vi "总氮总磷质控流程.vi"(0 "队列输入TP":refnum<queue>, 5 "总氮量程切换":enum32{"H", "L", "AUTO"}(ring)=enum."AUTO", 7 "总磷量程切换":enum32{"H", "L", "AUTO"}(ring)=enum."AUTO", 9 "总磷":bool, 11 "总氮":bool) -> (4 "布尔":bool, 6 "总磷中断报警":bool, 8 "总氮中断报警":bool)   [LabVIEW 2016, in "质控单元.lvlib"]
panel:
  out "总磷":bool
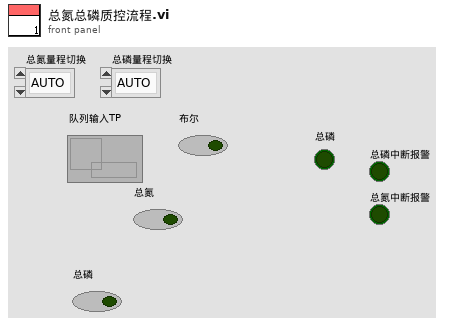
[diagram p1: front panel]
types:
  T1 = enum16{"待机", "启动氨氮水样", "氨氮测量中", "启动氨氮加标", "启动氨氮加标回收", "氨氮加标回收测量中", "启动总氮水样", "总氮测量中", "启动总氮加标", "启动总氮加标回收", "总氮加标回收测量中", "启动总磷水样", "总磷水样测量中", "启动总磷加标", "启动总磷加标回收", "总磷加标回收测量中", "结束"}
  T2 = cluster{"时间标识":timestamp, "设备":string, "日志信息":string}
  T3 = cluster{"站号":u16, "量程切换":enum32{"H", "L", "AUTO"}, "控制命令":enum16{"启动测量", "标样核查", "零点核查", "跨度核查", "空白测试", "平行样测试", "加标回收", "空白校准", "标样校准", "初始化（清洗）", "停止测试", "仪器重启", "校时", "模式设置", "测量间隔设置"}, "模式设置":enum16{"待机", "连续模式", "周期模式", "定点模式", "受控模式", "手动模式"}, "测量间隔":u16}
  T4 = cluster{"系统时间":timestamp, "工作状态":enum16{"空闲", "水样测试", "标样核查", "零点核查", "跨度核查", "空白测试", "平行样测试", "加标回收", "空白校准", "标样校准", "初始化（清洗）"}, "测量模式":enum16{"待机", "连续模式", "周期模式", "定点模式", "受控模式", "手动模式"}, "告警代码":enum16{"无告警", "缺试剂告警", "缺水样告警", "缺蒸馏水告警", "缺标液告警", "仪表漏液告警", "标定异常告警", "超量程告警", "加热异常", "低试剂预警", "超上限告警", "超下限告警", "仪表内部其他异常", "滴定异常告警", "电极异常告警", "量程切换告警", "参数设置告警", "PH电极电位异常", "电导率电极异常", "浊度光度异常", "溶解氧电极异常", "溶解氧光强异常", "温度异常告警", "PH异常告警", "溶解氧异常告警", "电导率异常告警", "浊度异常告警", "叶绿素异常告警", "藻密度异常告警", "蓝绿藻异常告警", "ORP异常告警", "氨氮异常告警", "清洁刷异常告警", "SD卡异常告警", "蓝牙异常告警", "Wifi异常告警", "流程异常告警"}, "故障代码":enum16{"无故障", "电机故障", "温度故障", "通讯故障", "滴定故障"}, "日志代码":u16, "软件版本":u16, "F0":sgl, "F1":sgl, "F2":sgl, "F3":sgl, "T":sgl, "H":sgl, "id":u16, "flowid":u16, "量程":u16}
  T5 = enum16{"空闲", "水样测试", "标样核查", "零点核查", "跨度核查", "空白测试", "平行样测试", "加标回收", "空白校准", "标样校准", "初始化（清洗）"}
  T6 = cluster{"因子编码":u32, "单位":u16, "标样参考值":sgl, "水样数据时间":timestamp, "水样实测值":sgl, "水样数据标识":string, "标样数据时间":timestamp, "标样实测值":sgl, "标样数据标识":string, "空白数据时间":timestamp, "空白实测值":sgl, "空白数据标识":string, "零点核查数据时间":timestamp, "零点核查实测值":sgl, "零点核查数据标识":string, "跨度核查数据时间":timestamp, "跨度核查实测值":sgl, "跨度核查数据标识":string, "加标回收数据时间":timestamp, "加标回收实测值":sgl, "加标回收数据标识":string, "平行样数据时间":timestamp, "平行样实测值":sgl, "平行样数据标识":string}
  T7 = cluster{"量程":dbl, "检出限":dbl, "加标前水样浓度":dbl, "加标后水样浓度":dbl, "加标水杯定容体积":dbl, "加标母液浓度":dbl, "加标体积":dbl, "加标回收率":dbl}
  T8 = cluster{"因子编码":u32, "单位":u16, "标样参考值":sgl, "水样数据时间":timestamp, "水样实测值":sgl, "水样数据标识":string, "标样数据时间":timestamp, "标样实测值":sgl, "标样数据标识":string, "空白数据时间":timestamp, "空白实测值":sgl, "空白数据标识":string, "零点核查数据时间":timestamp, "零点核查实测值":sgl, "零点核查数据标识":string, "跨度核查数据时间":timestamp, "跨度核查实测值":sgl, "跨度核查数据标识":string, "加标回收数据时间":timestamp, "加标回收实测值":sgl, "加标回收数据标识":string, "平行样数据时间":timestamp, "平行样实测值":sgl, "平行样数据标识":string, "F0":sgl, "F1":sgl, "F2":sgl, "F3":sgl, "F4":sgl, "F5":sgl, "F6":sgl, "F7":sgl, "温度":sgl, "湿度":sgl, "X值":sgl}
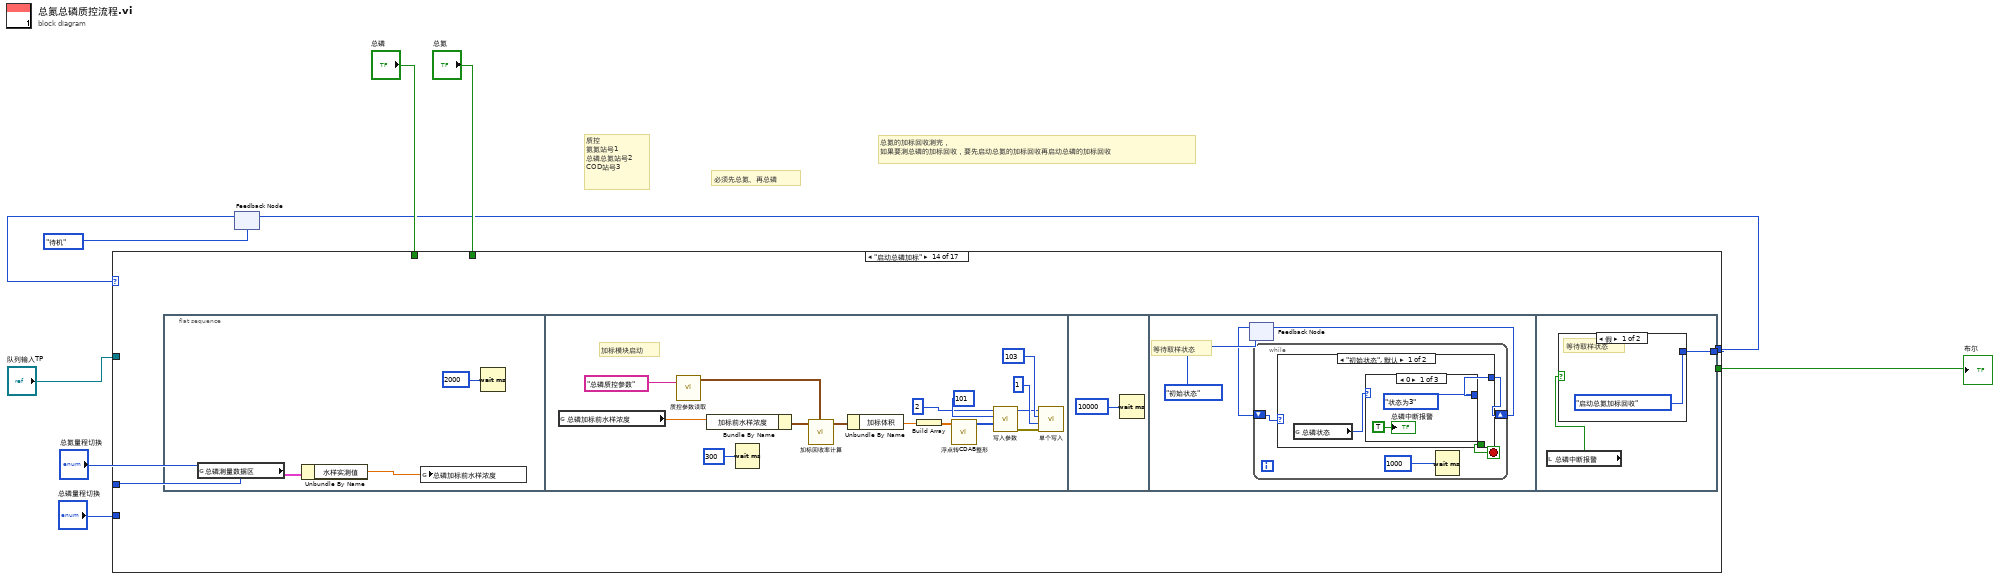
[diagram p0: block diagram]
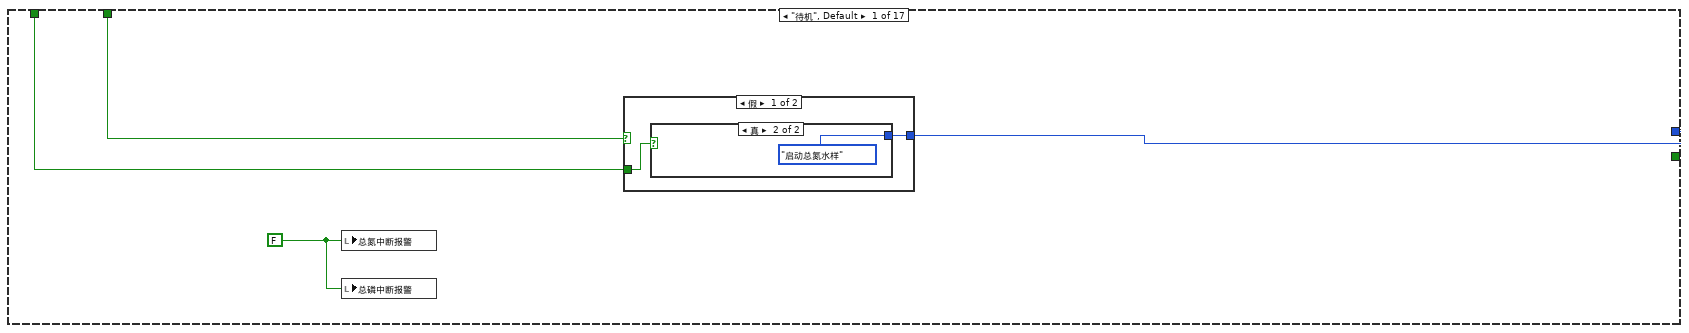
[diagram p2: hidden frame]
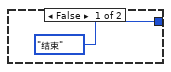
[diagram p3: hidden frame]
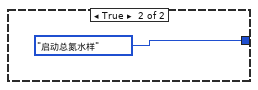
[diagram p4: hidden frame]
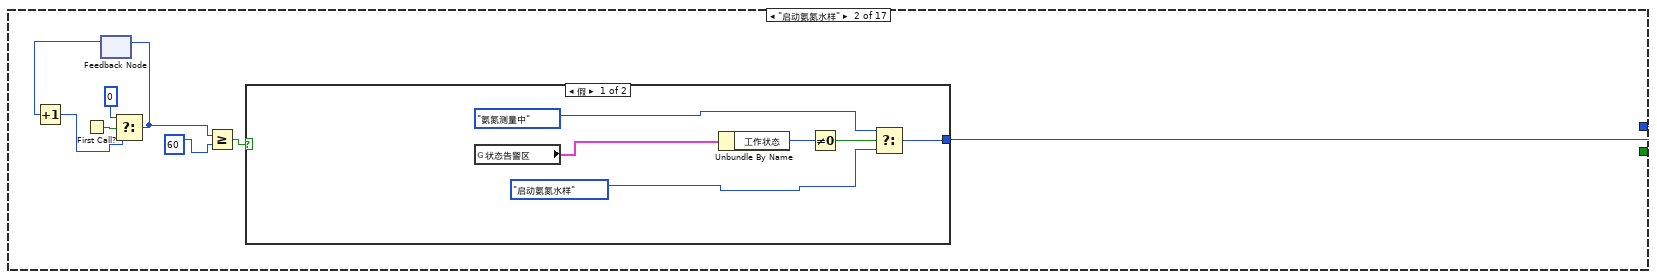
[diagram p5: hidden frame]
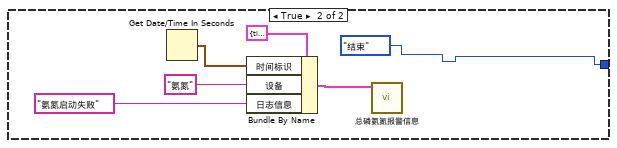
[diagram p6: hidden frame]
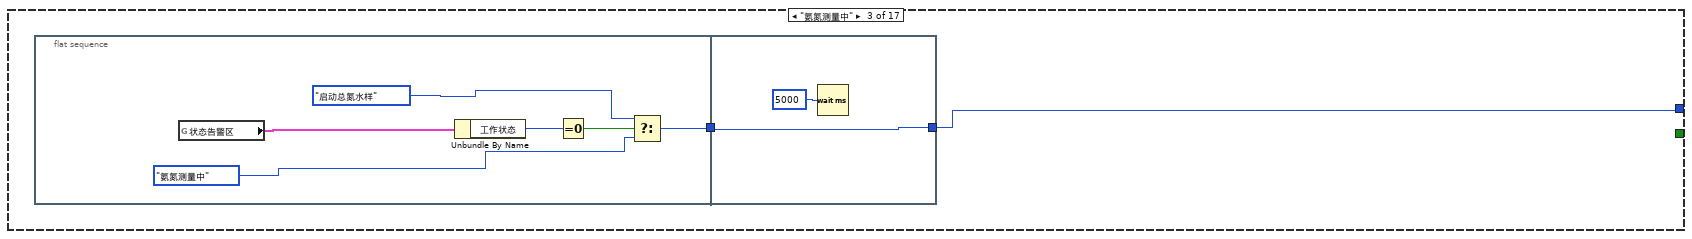
[diagram p7: hidden frame]
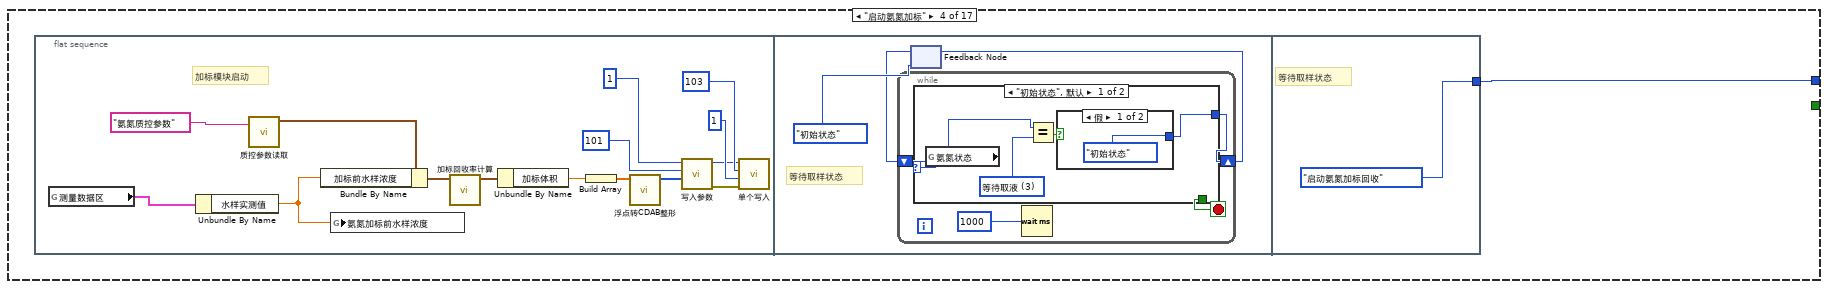
[diagram p8: hidden frame]
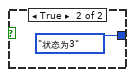
[diagram p9: hidden frame]
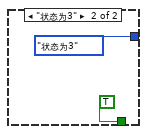
[diagram p10: hidden frame]
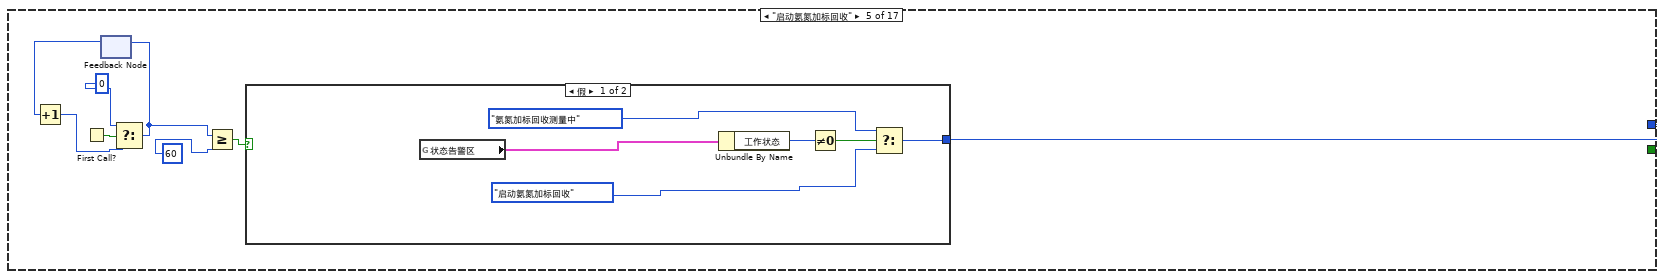
[diagram p11: hidden frame]
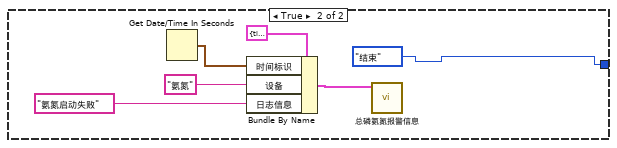
[diagram p12: hidden frame]
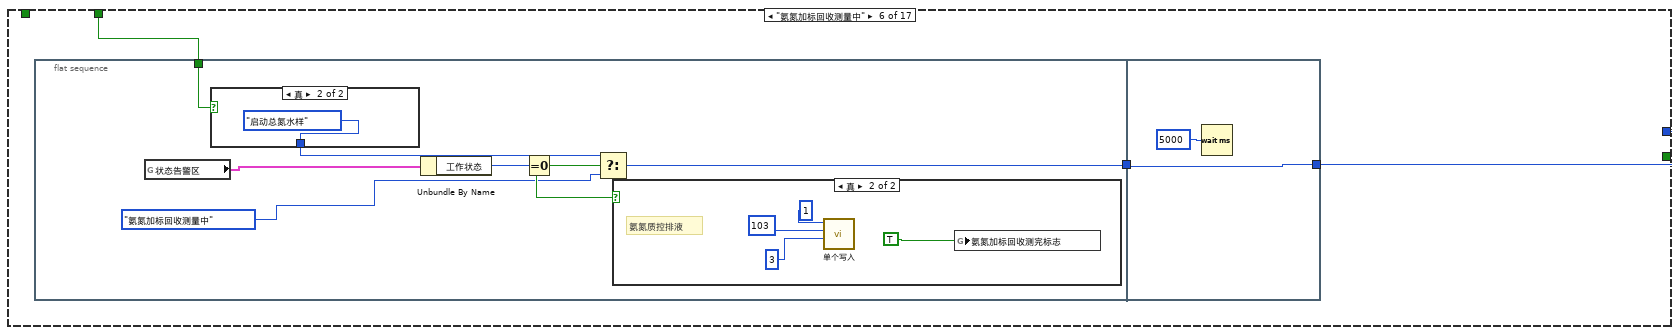
[diagram p13: hidden frame]
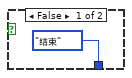
[diagram p14: hidden frame]
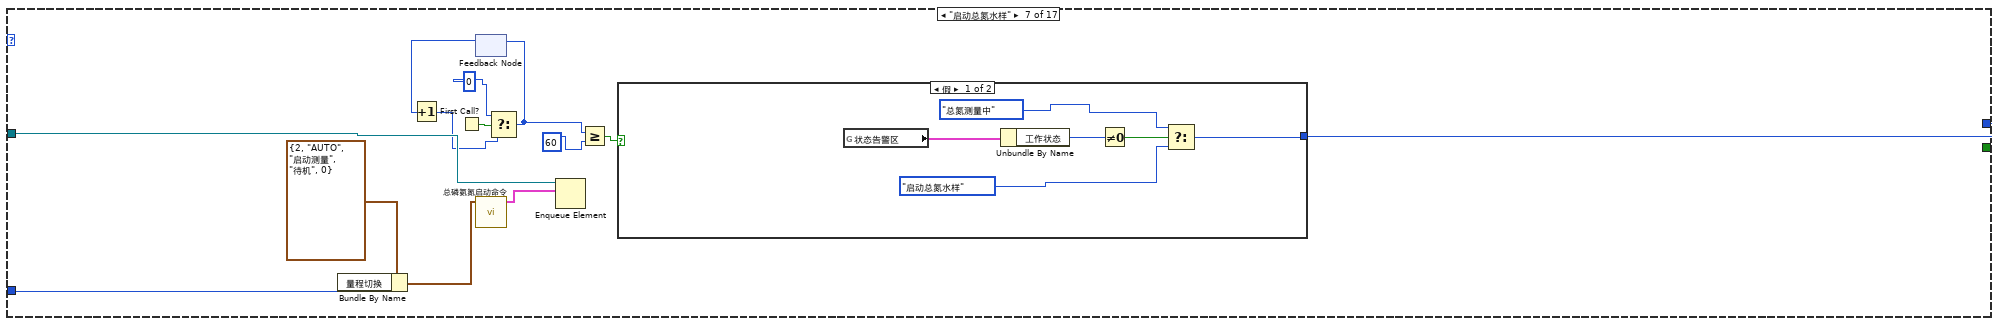
[diagram p16: hidden frame]
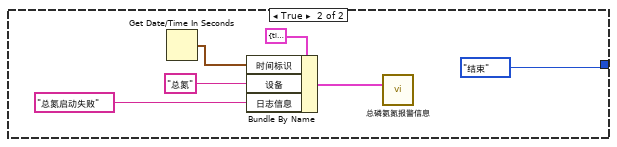
[diagram p17: hidden frame]
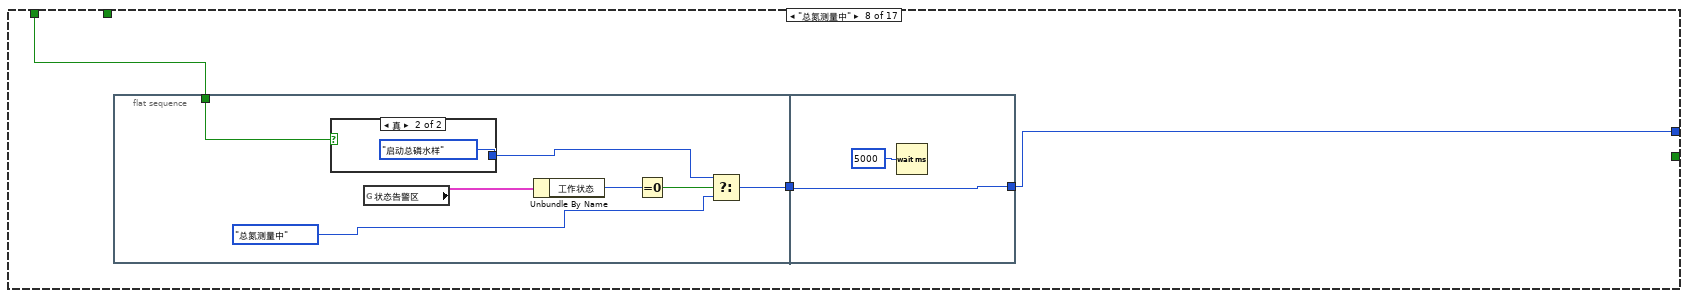
[diagram p18: hidden frame]
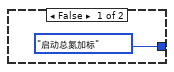
[diagram p19: hidden frame]
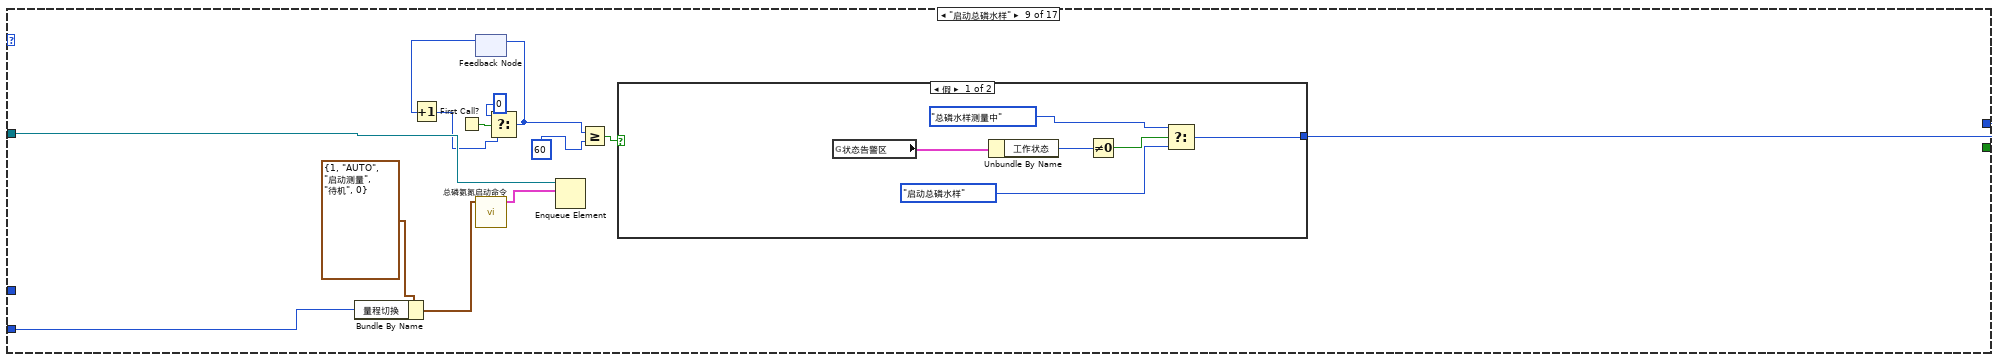
[diagram p20: hidden frame]
diagram:
  # "总氮的加标回收测完，\n如果要测总磷的加标回收，要先启动总氮的加标回收再启动总磷的加标回收"
  # "质控\n氨氮站号1   \n总磷总氮站号2\nCOD站号3"
  # "必须先总氮、再总磷"
  n1 = feedback #1(T1."待机") -> (w5:T1)
  n2 = case shown="\"启动总磷加标\"" w5 {
    tunnel: [w13 w26 w40 w49 w80 w100 w129 w144 w168 w184 w196 w238 w261 w290 w334 w356 T1."结束"] -> w3
    tunnel: "队列输入TP" -> [_ _ _ _ _ _ w130 _ w169 _ _ w240 _ _ w335 _ _]
    tunnel: [_ _ _ _ _ _ _ _ _ _ _ _ _ _ _ _ TRUE] -> w8
    tunnel: "总磷" -> [w12 _ _ _ _ _ _ w143 _ _ _ _ w262 _ _ _ _]
    tunnel: "总氮" -> [w11 _ _ _ _ w101 _ _ _ w182 _ _ w260 _ _ _ _]
    tunnel: "总氮量程切换" -> [_ _ _ _ _ _ w118 _ _ _ _ w235 _ _ _ _ _]
    tunnel: "总磷量程切换" -> [_ _ _ _ _ _ _ _ w157 _ _ _ _ _ w330 _ _]
    frame "待机", Default {
      w10 = FALSE ("总氮中断报警")
      n3 = local write "总氮中断报警"(w10) -> ()
      n4 = local write "总磷中断报警"(w10) -> ()
      n5 = case shown="假" w11 {
        tunnel: w12 -> [w14 _]
        tunnel: [w15 T1."启动总氮水样"] -> w13
        frame False {
          n6 = case shown="真" w14 {
            tunnel: [T1."结束" T1."启动总氮水样"] -> w15
            frame False {
            }
            frame True {
            }
          }
        }
        frame True {
        }
      }
    }
    frame "启动氨氮水样" {
      n7 = First Call?() -> (First Call?: T/F=w24:bool)
      n8 = feedback #2() -> (w23:i32)  [unwired: 1 in]
      n9 = Increment(x=w23) -> (x+1=w22:i32)
      n10 = Select(t=0, s=w24, f=w22) -> (s? t:f=w21:i32)
      n11 = feedback-in #2(w21) -> ()
      n12 = Greater Or Equal?(x=w21, y=60) -> (x >= y?=w19:bool)
      n13 = case shown="假" w19 {
        tunnel: [w30 T1."结束"] -> w26
        frame False {
          n14 = global read "VAR总磷氨氮全局变量.vi" "状态告警区"() -> (w27:T4)
          n15 = Unbundle By Name(w27) -> ("工作状态"=w32:T5)
          n16 = Not Equal To 0?(x=w32) -> (x != 0?=w31:bool)
          n17 = Select(t=T1."氨氮测量中", s=w31, f=T1."启动氨氮水样") -> (s? t:f=w30:T1)
        }
        frame True {
          n18 = Get Date/Time In Seconds() -> (seconds since 1Jan1904=w38:timestamp)
          n19 = Bundle By Name(cluster=T2 {"时间标识"=timestamp(0 s since 1904-01-01), "设备"="", "日志信息"=""} ("data in"), "时间标识"=w38, "设备"="氨氮", "日志信息"="氨氮启动失败") -> (w34:T2)
          n20 = call "总磷氨氮报警信息.vi"("data in"=w34) -> ()  [unwired: 11 in]
        }
      }
    }
    frame "氨氮测量中" {
      n21 = flat-sequence {
        tunnel: [w45] -> w39
        tunnel: [w48] -> w40
        tunnel: w39 -> [w48]
        frame #0 {
          n22 = global read "VAR总磷氨氮全局变量.vi" "状态告警区"() -> (w41:T4)
          n23 = Unbundle By Name(w41) -> ("工作状态"=w46:T5)
          n24 = Equal To 0?(x=w46) -> (x = 0?=w44:bool)
          n25 = Select(t=T1."启动总氮水样", s=w44, f=T1."氨氮测量中") -> (s? t:f=w45:T1)
        }
        frame #1 {
          n26 = Wait (ms)(milliseconds to wait=u32 5000 ("等待时间（毫秒）")) -> ()  [unwired: 1 out]
        }
      }
    }
    frame "启动氨氮加标" {
      n27 = flat-sequence {
        tunnel: [T1."启动氨氮加标回收"] -> w49
        frame #0 {
          w53 = u16 1 ("value")
          # "加标模块启动"
          n28 = global read "VAR总磷氨氮全局变量.vi" "测量数据区"() -> (w50:T6)
          n29 = Unbundle By Name(w50) -> ("水样实测值"=w51:sgl)
          n30 = call "质控参数读取.vi"("section"="氨氮质控参数") -> ("参数"=w61:T7)  [unwired: 9 in, 1 out]
          n31 = Bundle By Name(cluster=w61, "加标前水样浓度"=w51) -> (w62:T7)
          n32 = global write "水样浓度全局.vi" "氨氮加标前水样浓度"(w51) -> ()
          n33 = call "加标回收率计算.vi"("参数"=w62) -> ("参数 out"=w60:T7)  [unwired: 10 in]
          n34 = Unbundle By Name(w60) -> ("加标体积"=w52:dbl)
          n35 = Build Array(w52) -> (w59:dbl[])
          n36 = call "浮点转CDAB整形.vi"("浮点数"=w59) -> ("CDAB整形输出"=w54:u16[])  [unwired: 10 in]
          n37 = call "写入参数.vi"("values"=w54, "starting address"=u16 101, "Slave ID"=w53) -> ("error out"=w58:errorcluster)  [unwired: 8 in]
          n38 = call "单个写入.vi"("Error in"=w58, "value"=u16 1, "address"=u16 103, "Slave ID"=w53) -> ()  [unwired: 7 in, 1 out]
        }
        frame #1 {
          # "等待取样状态"
          n39 = feedback #3(enum16{"初始状态", "状态为3"}."初始状态") -> (w65:enum16{"初始状态", "状态为3"})
          n40 = while {
            shift-right: [w69] -> w64
            shift-left: w65 -> [w70]
            stop <- w68 stop-if-true
            n41 = case shown="\"初始状态\", 默认" w70 {
              tunnel: [w72 enum16{"初始状态", "状态为3"}."状态为3"] -> w69
              tunnel: [_ TRUE] -> w68
              frame "初始状态", Default {
                w71 = u16 3 items=["待机", "润洗", "进样", "等待取液", "排液"] ("氨氮状态")
                n42 = global read "氨氮加标回收状态全局变量.vi" "氨氮状态"() -> (w74:u16)
                n43 = Equal?(x=w74, y=w71) -> (x = y?=w73:bool)
                n44 = case shown="假" w73 {
                  tunnel: [enum16{"初始状态", "状态为3"}."初始状态" enum16{"初始状态", "状态为3"}."状态为3"] -> w72
                  frame False {
                  }
                  frame True {
                  }
                }
              }
              frame "状态为3" {
              }
            }
            n45 = Wait (ms)(milliseconds to wait=u32 1000 ("等待时间（毫秒）")) -> ()  [unwired: 1 out]
          }
          n46 = feedback-in #3(w64) -> ()
        }
        frame #2 {
          # "等待取样状态"
        }
      }
    }
    frame "启动氨氮加标回收" {
      n47 = First Call?() -> (First Call?: T/F=w86:bool)
      n48 = feedback #4() -> (w85:i32)  [unwired: 1 in]
      n49 = Increment(x=w85) -> (x+1=w84:i32)
      n50 = Select(t=0, s=w86, f=w84) -> (s? t:f=w83:i32)
      n51 = feedback-in #4(w83) -> ()
      n52 = Greater Or Equal?(x=w83, y=60) -> (x >= y?=w81:bool)
      n53 = case shown="假" w81 {
        tunnel: [w91 T1."结束"] -> w80
        frame False {
          n54 = global read "VAR总磷氨氮全局变量.vi" "状态告警区"() -> (w88:T4)
          n55 = Unbundle By Name(w88) -> ("工作状态"=w93:T5)
          n56 = Not Equal To 0?(x=w93) -> (x != 0?=w92:bool)
          n57 = Select(t=T1."氨氮加标回收测量中", s=w92, f=T1."启动氨氮加标回收") -> (s? t:f=w91:T1)
        }
        frame True {
          n58 = Get Date/Time In Seconds() -> (seconds since 1Jan1904=w99:timestamp)
          n59 = Bundle By Name(cluster=T2 {"时间标识"=timestamp(0 s since 1904-01-01), "设备"="", "日志信息"=""} ("data in"), "时间标识"=w99, "设备"="氨氮", "日志信息"="氨氮启动失败") -> (w95:T2)
          n60 = call "总磷氨氮报警信息.vi"("data in"=w95) -> ()  [unwired: 11 in]
        }
      }
    }
    frame "氨氮加标回收测量中" {
      n61 = flat-sequence {
        tunnel: [w108] -> w102
        tunnel: w101 -> [w105]
        tunnel: [w117] -> w100
        tunnel: w102 -> [w117]
        frame #0 {
          n62 = global read "VAR总磷氨氮全局变量.vi" "状态告警区"() -> (w103:T4)
          n63 = case shown="真" w105 {
            tunnel: [T1."结束" T1."启动总氮水样"] -> w107
            frame False {
            }
            frame True {
            }
          }
          n64 = Unbundle By Name(w103) -> ("工作状态"=w109:T5)
          n65 = Equal To 0?(x=w109) -> (x = 0?=w106:bool)
          n66 = Select(t=w107, s=w106, f=T1."氨氮加标回收测量中") -> (s? t:f=w108:T1)
          n67 = case shown="真" w106 {
            frame False {
            }
            frame True {
              # "氨氮质控排液"
              n68 = call "单个写入.vi"("value"=u16 3, "address"=u16 103, "Slave ID"=u8 1) -> ()  [unwired: 8 in, 1 out]
              n69 = global write "质控测完标志全局 1.vi" "氨氮加标回收测完标志"(TRUE) -> ()
            }
          }
        }
        frame #1 {
          n70 = Wait (ms)(milliseconds to wait=u32 5000 ("等待时间（毫秒）")) -> ()  [unwired: 1 out]
        }
      }
    }
    frame "启动总氮水样" {
      n71 = Bundle By Name(cluster=T3 {"站号"=2, "量程切换"=enum."AUTO", "控制命令"=enum."启动测量", "模式设置"=enum."待机", "测量间隔"=0} ("参数"), "量程切换"=w118) -> (w119:T3)
      n72 = First Call?() -> (First Call?: T/F=w127:bool)
      n73 = feedback #5() -> (w126:i32)  [unwired: 1 in]
      n74 = Increment(x=w126) -> (x+1=w125:i32)
      n75 = call "总磷氨氮启动命令.vi"("参数"=w119) -> ("启动命令"=w121:cluster{"命令":string, "data":variant})  [unwired: 10 in]
      n76 = Select(t=0, s=w127, f=w125) -> (s? t:f=w124:i32)
      n77 = feedback-in #5(w124) -> ()
      n78 = Enqueue Element(queue=w130, element=w121) -> ()  [unwired: 2 in, 3 out]
      n79 = Greater Or Equal?(x=w124, y=60) -> (x >= y?=w122:bool)
      n80 = case shown="假" w122 {
        tunnel: [w133 T1."结束"] -> w129
        frame False {
          n81 = global read "VAR总磷氨氮全局变量.vi" "状态告警区"() -> (w134:T4)
          n82 = Unbundle By Name(w134) -> ("工作状态"=w135:T5)
          n83 = Not Equal To 0?(x=w135) -> (x != 0?=w136:bool)
          n84 = Select(t=T1."总氮测量中", s=w136, f=T1."启动总氮水样") -> (s? t:f=w133:T1)
        }
        frame True {
          n85 = Get Date/Time In Seconds() -> (seconds since 1Jan1904=w142:timestamp)
          n86 = Bundle By Name(cluster=T2 {"时间标识"=timestamp(0 s since 1904-01-01), "设备"="", "日志信息"=""} ("data in"), "时间标识"=w142, "设备"="总氮", "日志信息"="总氮启动失败") -> (w138:T2)
          n87 = call "总磷氨氮报警信息.vi"("data in"=w138) -> ()  [unwired: 11 in]
        }
      }
    }
    frame "总氮测量中" {
      n88 = flat-sequence {
        tunnel: [w150] -> w145
        tunnel: w143 -> [w146]
        tunnel: [w156] -> w144
        tunnel: w145 -> [w156]
        frame #0 {
          n89 = case shown="真" w146 {
            tunnel: [T1."启动总氮加标" T1."启动总磷水样"] -> w148
            frame False {
            }
            frame True {
            }
          }
          n90 = global read "VAR总磷氨氮全局变量.vi" "状态告警区"() -> (w151:T4)
          n91 = Unbundle By Name(w151) -> ("工作状态"=w152:T5)
          n92 = Equal To 0?(x=w152) -> (x = 0?=w149:bool)
          n93 = Select(t=w148, s=w149, f=T1."总氮测量中") -> (s? t:f=w150:T1)
        }
        frame #1 {
          n94 = Wait (ms)(milliseconds to wait=u32 5000 ("等待时间（毫秒）")) -> ()  [unwired: 1 out]
        }
      }
    }
    frame "启动总磷水样" {
      n95 = Bundle By Name(cluster=T3 {"站号"=1, "量程切换"=enum."AUTO", "控制命令"=enum."启动测量", "模式设置"=enum."待机", "测量间隔"=0} ("参数"), "量程切换"=w157) -> (w158:T3)
      n96 = First Call?() -> (First Call?: T/F=w166:bool)
      n97 = feedback #6() -> (w165:i32)  [unwired: 1 in]
      n98 = Increment(x=w165) -> (x+1=w164:i32)
      n99 = call "总磷氨氮启动命令.vi"("参数"=w158) -> ("启动命令"=w160:cluster{"命令":string, "data":variant})  [unwired: 10 in]
      n100 = Select(t=0, s=w166, f=w164) -> (s? t:f=w163:i32)
      n101 = feedback-in #6(w163) -> ()
      n102 = Enqueue Element(queue=w169, element=w160) -> ()  [unwired: 2 in, 3 out]
      n103 = Greater Or Equal?(x=w163, y=60) -> (x >= y?=w161:bool)
      n104 = case shown="假" w161 {
        tunnel: [w172 T1."结束"] -> w168
        frame False {
          n105 = global read "VAR总磷氨氮全局变量.vi" "状态告警区"() -> (w173:T4)
          n106 = Unbundle By Name(w173) -> ("工作状态"=w174:T5)
          n107 = Not Equal To 0?(x=w174) -> (x != 0?=w175:bool)
          n108 = Select(t=T1."总磷水样测量中", s=w175, f=T1."启动总磷水样") -> (s? t:f=w172:T1)
        }
        frame True {
          n109 = Get Date/Time In Seconds() -> (seconds since 1Jan1904=w181:timestamp)
          n110 = Bundle By Name(cluster=T2 {"时间标识"=timestamp(0 s since 1904-01-01), "设备"="", "日志信息"=""} ("data in"), "时间标识"=w181, "设备"="总磷", "日志信息"="总磷启动失败") -> (w177:T2)
          n111 = call "总磷氨氮报警信息.vi"("data in"=w177) -> ()  [unwired: 11 in]
        }
      }
    }
    frame "总磷水样测量中" {
      n112 = flat-sequence {
        tunnel: [w189] -> w183
        tunnel: w182 -> [w186]
        tunnel: [w195] -> w184
        tunnel: w183 -> [w195]
        frame #0 {
          n113 = case shown="真" w186 {
            tunnel: [T1."启动总磷加标" T1."启动总氮加标"] -> w187
            frame False {
            }
            frame True {
            }
          }
          n114 = global read "VAR总磷氨氮全局变量.vi" "状态告警区"() -> (w190:T4)
          n115 = Unbundle By Name(w190) -> ("工作状态"=w191:T5)
          n116 = Equal To 0?(x=w191) -> (x = 0?=w188:bool)
          n117 = Select(t=w187, s=w188, f=T1."总磷水样测量中") -> (s? t:f=w189:T1)
        }
        frame #1 {
          n118 = Wait (ms)(milliseconds to wait=u32 7000 ("等待时间（毫秒）")) -> ()  [unwired: 1 out]
        }
      }
    }
    frame "启动总氮加标" {
      n119 = flat-sequence {
        tunnel: [w232] -> w196
        frame #0 {
          n120 = global read "VAR总磷氨氮全局变量.vi" "总氮测量数据区"() -> (w199:T8)
          n121 = Unbundle By Name(w199) -> ("水样实测值"=w198:sgl)
          n122 = global write "水样浓度全局.vi" "总氮加标前水样浓度"(w198) -> ()
          n123 = Wait (ms)(milliseconds to wait=u32 2000 ("等待时间（毫秒）")) -> ()  [unwired: 1 out]
        }
        frame #1 {
          w204 = u16 2 ("value")
          # "加标模块启动"
          n124 = global read "水样浓度全局.vi" "总氮加标前水样浓度"() -> (w201:dbl)
          n125 = call "质控参数读取.vi"("section"="总氮质控参数") -> ("参数"=w202:T7)  [unwired: 9 in, 1 out]
          n126 = Bundle By Name(cluster=w202, "加标前水样浓度"=w201) -> (w212:T7)
          n127 = Wait (ms)(milliseconds to wait=u32 300 ("等待时间（毫秒）")) -> ()  [unwired: 1 out]
          n128 = call "加标回收率计算.vi"("参数"=w212) -> ("参数 out"=w211:T7)  [unwired: 10 in]
          n129 = Unbundle By Name(w211) -> ("加标体积"=w203:dbl)
          n130 = Build Array(w203) -> (w210:dbl[])
          n131 = call "浮点转CDAB整形.vi"("浮点数"=w210) -> ("CDAB整形输出"=w205:u16[])  [unwired: 10 in]
          n132 = call "写入参数.vi"("values"=w205, "starting address"=u16 101, "Slave ID"=w204) -> ("error out"=w209:errorcluster)  [unwired: 8 in]
          n133 = call "单个写入.vi"("Error in"=w209, "value"=u16 1, "address"=u16 103, "Slave ID"=w204) -> ()  [unwired: 7 in, 1 out]
        }
        frame #2 {
          n134 = Wait (ms)(milliseconds to wait=u32 10000 ("等待时间（毫秒）")) -> ()  [unwired: 1 out]
        }
        frame #3 {
          # "等待取样状态"
          n135 = feedback #7(enum16{"初始状态", "状态为3"}."初始状态") -> (w216:enum16{"初始状态", "状态为3"})
          n136 = while {
            shift-right: [w220] -> w215
            shift-left: w216 -> [w221]
            stop <- w219 stop-if-true
            n137 = case shown="\"初始状态\", 默认" w221 {
              tunnel: [w223 enum16{"初始状态", "状态为3"}."状态为3"] -> w220
              tunnel: [_ TRUE] -> w219
              frame "初始状态", Default {
                n138 = global read "氨氮加标回收状态全局变量.vi" "总氮状态"() -> (w222:u16)
                n139 = case shown="3" w222 {
                  tunnel: [enum16{"初始状态", "状态为3"}."状态为3" enum16{"初始状态", "状态为3"}."初始状态" enum16{"初始状态", "状态为3"}."状态为3"] -> w223
                  frame 0 {
                    "总氮中断报警" <- TRUE ("总氮中断报警")
                  }
                  frame 1, Default {
                  }
                  frame 3 {
                    n140 = local write "总氮中断报警"(FALSE ("总氮中断报警")) -> ()
                  }
                }
              }
              frame "状态为3" {
              }
            }
            n141 = Wait (ms)(milliseconds to wait=u32 1000 ("等待时间（毫秒）")) -> ()  [unwired: 1 out]
          }
          n142 = feedback-in #7(w215) -> ()
        }
        frame #4 {
          # "等待取样状态"
          n143 = local read "总氮中断报警"() -> (w231:bool)
          n144 = case shown="假" w231 {
            tunnel: [T1."启动总氮加标回收" T1."结束"] -> w232
            frame False {
            }
            frame True {
            }
          }
        }
      }
    }
    frame "启动总氮加标回收" {
      n145 = Bundle By Name(cluster=T3 {"站号"=2, "量程切换"=enum."AUTO", "控制命令"=enum."加标回收", "模式设置"=enum."待机", "测量间隔"=0} ("参数"), "量程切换"=w235) -> (w236:T3)
      n146 = First Call?() -> (First Call?: T/F=w246:bool)
      n147 = call "总磷氨氮启动命令.vi"("参数"=w236) -> ("启动命令"=w239:cluster{"命令":string, "data":variant})  [unwired: 10 in]
      n148 = feedback #8() -> (w245:i32)  [unwired: 1 in]
      n149 = Increment(x=w245) -> (x+1=w244:i32)
      n150 = Select(t=0, s=w246, f=w244) -> (s? t:f=w243:i32)
      n151 = feedback-in #8(w243) -> ()
      n152 = Enqueue Element(queue=w240, element=w239) -> ()  [unwired: 2 in, 3 out]
      n153 = Greater Or Equal?(x=w243, y=60) -> (x >= y?=w241:bool)
      n154 = case shown="假" w241 {
        tunnel: [w250 T1."结束"] -> w238
        frame False {
          n155 = global read "VAR总磷氨氮全局变量.vi" "状态告警区"() -> (w253:T4)
          n156 = Unbundle By Name(w253) -> ("工作状态"=w252:T5)
          n157 = Not Equal To 0?(x=w252) -> (x != 0?=w251:bool)
          n158 = Select(t=T1."总氮加标回收测量中", s=w251, f=T1."启动总氮加标回收") -> (s? t:f=w250:T1)
        }
        frame True {
          n159 = Get Date/Time In Seconds() -> (seconds since 1Jan1904=w259:timestamp)
          n160 = Bundle By Name(cluster=T2 {"时间标识"=timestamp(0 s since 1904-01-01), "设备"="", "日志信息"=""} ("data in"), "时间标识"=w259, "设备"="总氮", "日志信息"="总氮启动失败") -> (w255:T2)
          n161 = call "总磷氨氮报警信息.vi"("data in"=w255) -> ()  [unwired: 11 in]
        }
      }
    }
    frame "总氮加标回收测量中" {
      n162 = flat-sequence {
        tunnel: [w272] -> w263
        tunnel: w262 -> [w269]
        tunnel: w260 -> [w265]
        tunnel: [w289] -> w261
        tunnel: w263 -> [w289]
        frame #0 {
          n163 = case shown="真" w269 {
            tunnel: [T1."结束" w277] -> w271
            tunnel: w265 -> [_ w276]
            frame False {
            }
            frame True {
              n164 = case shown="真" w276 {
                tunnel: [T1."启动总磷加标回收" w280] -> w277
                frame False {
                }
                frame True {
                  n165 = local read "总磷"() -> (w279:bool)
                  n166 = case shown="真" w279 {
                    tunnel: [T1."启动总磷加标" T1."启动总磷加标回收"] -> w280
                    frame False {
                    }
                    frame True {
                    }
                  }
                }
              }
            }
          }
          n167 = global read "VAR总磷氨氮全局变量.vi" "状态告警区"() -> (w273:T4)
          n168 = Unbundle By Name(w273) -> ("工作状态"=w274:T5)
          n169 = local read "总磷"() -> (w267:bool)
          n170 = Equal To 0?(x=w274) -> (x = 0?=w270:bool)
          n171 = Not(x=w267) -> (.not. x?=w266:bool)
          n172 = And(x=w270, y=w266) -> (x .and. y?=w264:bool)
          n173 = Select(t=w271, s=w270, f=T1."总氮加标回收测量中") -> (s? t:f=w272:T1)
          n174 = case shown="真" w264 {
            frame False {
            }
            frame True {
              # "总氮质控排液"
              n175 = call "单个写入.vi"("value"=u16 3, "address"=u16 103, "Slave ID"=u8 2) -> ()  [unwired: 8 in, 1 out]
              n176 = global write "质控测完标志全局 1.vi" "总氮加标回收测完标志"(TRUE) -> ()
              n177 = Wait (ms)(milliseconds to wait=u32 180000 ("等待时间（毫秒）")) -> ()  [unwired: 1 out]
            }
          }
        }
        frame #1 {
          n178 = Wait (ms)(milliseconds to wait=u32 7000 ("等待时间（毫秒）")) -> ()  [unwired: 1 out]
        }
      }
    }
    frame "启动总磷加标" {
      n179 = flat-sequence {
        tunnel: [w327] -> w290
        frame #0 {
          n180 = global read "VAR总磷氨氮全局变量.vi" "总磷测量数据区"() -> (w293:T8)
          n181 = Unbundle By Name(w293) -> ("水样实测值"=w292:sgl)
          n182 = global write "水样浓度全局.vi" "总磷加标前水样浓度"(w292) -> ()
          n183 = Wait (ms)(milliseconds to wait=u32 2000 ("等待时间（毫秒）")) -> ()  [unwired: 1 out]
        }
        frame #1 {
          w298 = u16 2 ("value")
          # "加标模块启动"
          n184 = global read "水样浓度全局.vi" "总磷加标前水样浓度"() -> (w295:dbl)
          n185 = call "质控参数读取.vi"("section"="总磷质控参数") -> ("参数"=w296:T7)  [unwired: 9 in, 1 out]
          n186 = Bundle By Name(cluster=w296, "加标前水样浓度"=w295) -> (w306:T7)
          n187 = Wait (ms)(milliseconds to wait=u32 300 ("等待时间（毫秒）")) -> ()  [unwired: 1 out]
          n188 = call "加标回收率计算.vi"("参数"=w306) -> ("参数 out"=w305:T7)  [unwired: 10 in]
          n189 = Unbundle By Name(w305) -> ("加标体积"=w297:dbl)
          n190 = Build Array(w297) -> (w304:dbl[])
          n191 = call "浮点转CDAB整形.vi"("浮点数"=w304) -> ("CDAB整形输出"=w299:u16[])  [unwired: 10 in]
          n192 = call "写入参数.vi"("values"=w299, "starting address"=u16 101, "Slave ID"=w298) -> ("error out"=w303:errorcluster)  [unwired: 8 in]
          n193 = call "单个写入.vi"("Error in"=w303, "value"=u16 1, "address"=u16 103, "Slave ID"=w298) -> ()  [unwired: 7 in, 1 out]
        }
        frame #2 {
          n194 = Wait (ms)(milliseconds to wait=u32 10000 ("等待时间（毫秒）")) -> ()  [unwired: 1 out]
        }
        frame #3 {
          # "等待取样状态"
          n195 = feedback #9(enum16{"初始状态", "状态为3"}."初始状态") -> (w310:enum16{"初始状态", "状态为3"})
          n196 = while {
            shift-right: [w314] -> w309
            shift-left: w310 -> [w315]
            stop <- w313 stop-if-true
            n197 = case shown="\"初始状态\", 默认" w315 {
              tunnel: [w317 enum16{"初始状态", "状态为3"}."状态为3"] -> w314
              tunnel: [_ TRUE] -> w313
              frame "初始状态", Default {
                n198 = global read "氨氮加标回收状态全局变量.vi" "总磷状态"() -> (w316:u16)
                n199 = case shown="0" w316 {
                  tunnel: [enum16{"初始状态", "状态为3"}."状态为3" enum16{"初始状态", "状态为3"}."初始状态" enum16{"初始状态", "状态为3"}."状态为3"] -> w317
                  frame 0 {
                    "总磷中断报警" <- TRUE ("总磷中断报警")
                  }
                  frame 1, Default {
                  }
                  frame 3 {
                    n200 = local write "总磷中断报警"(FALSE ("总磷中断报警")) -> ()
                  }
                }
              }
              frame "状态为3" {
                "总磷" <- TRUE
              }
            }
            n201 = Wait (ms)(milliseconds to wait=u32 1000 ("等待时间（毫秒）")) -> ()  [unwired: 1 out]
          }
          n202 = feedback-in #9(w309) -> ()
        }
        frame #4 {
          n203 = local read "总磷中断报警"() -> (w326:bool)
          n204 = case shown="假" w326 {
            tunnel: [T1."启动总氮加标回收" T1."结束"] -> w327
            frame False {
              # "等待取样状态"
            }
            frame True {
            }
          }
        }
      }
    }
    frame "启动总磷加标回收" {
      n205 = Bundle By Name(cluster=T3 {"站号"=1, "量程切换"=enum."AUTO", "控制命令"=enum."加标回收", "模式设置"=enum."待机", "测量间隔"=0} ("参数"), "量程切换"=w330) -> (w331:T3)
      n206 = First Call?() -> (First Call?: T/F=w342:bool)
      n207 = feedback #10() -> (w341:i32)  [unwired: 1 in]
      n208 = Increment(x=w341) -> (x+1=w340:i32)
      n209 = call "总磷氨氮启动命令.vi"("参数"=w331) -> ("启动命令"=w336:cluster{"命令":string, "data":variant})  [unwired: 10 in]
      n210 = Select(t=0, s=w342, f=w340) -> (s? t:f=w339:i32)
      n211 = feedback-in #10(w339) -> ()
      n212 = Enqueue Element(queue=w335, element=w336) -> ()  [unwired: 2 in, 3 out]
      n213 = Greater Or Equal?(x=w339, y=60) -> (x >= y?=w337:bool)
      n214 = case shown="假" w337 {
        tunnel: [w346 T1."结束"] -> w334
        frame False {
          n215 = global read "VAR总磷氨氮全局变量.vi" "状态告警区"() -> (w347:T4)
          n216 = Unbundle By Name(w347) -> ("工作状态"=w348:T5)
          n217 = Not Equal To 0?(x=w348) -> (x != 0?=w349:bool)
          n218 = Select(t=T1."总磷加标回收测量中", s=w349, f=T1."启动总磷加标回收") -> (s? t:f=w346:T1)
        }
        frame True {
          n219 = Get Date/Time In Seconds() -> (seconds since 1Jan1904=w355:timestamp)
          n220 = Bundle By Name(cluster=T2 {"时间标识"=timestamp(0 s since 1904-01-01), "设备"="", "日志信息"=""} ("data in"), "时间标识"=w355, "设备"="总磷", "日志信息"="总磷启动失败") -> (w351:T2)
          n221 = call "总磷氨氮报警信息.vi"("data in"=w351) -> ()  [unwired: 11 in]
        }
      }
      n222 = local write "总磷"(FALSE ("总磷")) -> ()
    }
    frame "总磷加标回收测量中" {
      n223 = flat-sequence {
        tunnel: [w361] -> w357
        tunnel: [w369] -> w356
        tunnel: w357 -> [w369]
        frame #0 {
          n224 = global read "VAR总磷氨氮全局变量.vi" "状态告警区"() -> (w362:T4)
          n225 = Unbundle By Name(w362) -> ("工作状态"=w363:T5)
          n226 = Equal To 0?(x=w363) -> (x = 0?=w360:bool)
          n227 = Select(t=T1."结束", s=w360, f=T1."总磷加标回收测量中") -> (s? t:f=w361:T1)
          n228 = case shown="真" w360 {
            frame False {
            }
            frame True {
              # "总磷质控排液"
              n229 = global write "质控测完标志全局 1.vi" "总磷加标回收测完标志"(TRUE) -> ()
              n230 = call "单个写入.vi"("value"=u16 3, "address"=u16 103, "Slave ID"=u8 2) -> ()  [unwired: 8 in, 1 out]
            }
          }
        }
        frame #1 {
          n231 = Wait (ms)(milliseconds to wait=u32 5000 ("等待时间（毫秒）")) -> ()  [unwired: 1 out]
        }
      }
    }
    frame "结束" {
    }
  }
  "布尔" <- w8
  n232 = feedback-in #1(w3) -> ()
